vi "Convert Plot Interpolation (PN to List).vi"(8 "Error In":errorcluster, 11 "Plot Interpolation (PN)":u8) -> (0 "Error Out":errorcluster, 3 "Plot Interpolation (List)":T1)   [LabVIEW 2021, in "Graphs.lvlib"]
uses:
  LabVIEW Plot Interpolation.ctl
  Graphs.lvlib
panel:
  # "see the License on the block diagram (Ctrl+E or Window:Show Block Diagram)"
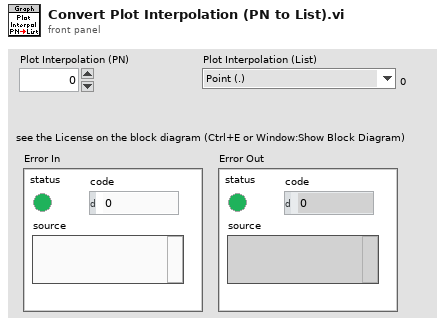
[diagram p1: front panel]
types:
  T1 = typedef "Graphs.lvlib/LabVIEW Plot Interpolation.ctl" = enum16{"Point (.)", "Stepwise Right (--.)", "Line + Point (\\. /)", "Stepwise Left (.--)", "Stepwise Centered (-.-)", "Stepwise Vertical (|.|)", "Line (-)", "Use Previous Plot's Style"}
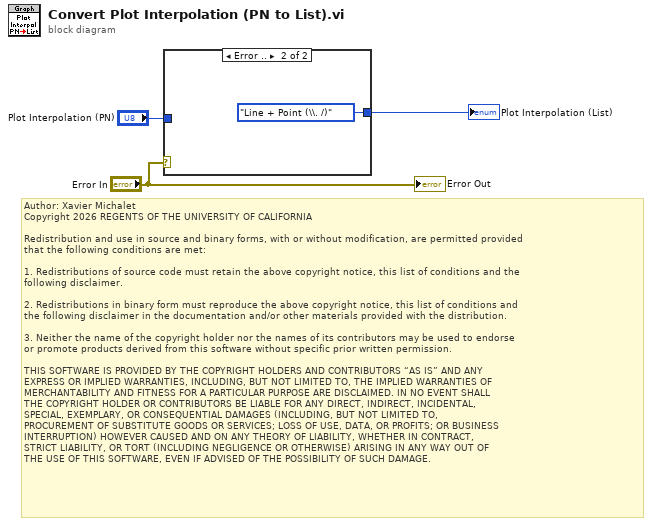
[diagram p0: block diagram]
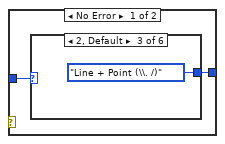
[diagram p2: hidden frame]
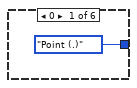
[diagram p3: hidden frame]
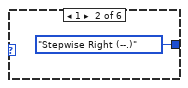
[diagram p4: hidden frame]
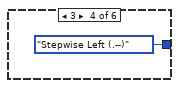
[diagram p5: hidden frame]
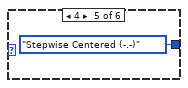
[diagram p6: hidden frame]
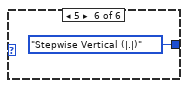
[diagram p7: hidden frame]
diagram:
  # "Author: Xavier Michalet\nCopyright 2026 REGENTS OF THE UNIVERSITY OF CALIFORNIA\n\nRedistribution and use in source and binary forms, with or without modification, are permitted provided\nthat the following conditions are met:\n\n1. Redistributions of source code must retain the above copyright notice, this list of conditions and the\nfollowing disclaimer.\n\n2. Redistributions in binary form must reproduce the above copyright notice, this list of conditions and\nthe following disclaimer in the documentation and/or other materials provided with the distribution.\n\n3. Neither the name of the copyright holder nor the names of its contributors may be used to endorse \nor promote products derived from this software without specific prior written permission.\n\nTHIS SOFTWARE IS PROVIDED BY THE COPYRIGHT HOLDERS AND CONTRIBUTORS “AS IS” AND ANY \nEXPRESS OR IMPLIED WARRANTIES, INCLUDING, BUT NOT LIMITED TO, THE IMPLIED WARRANTIES OF\nMERCHANTABILITY AND FITNESS FOR A PARTICULAR PURPOSE ARE DISCLAIMED. IN NO EVENT SHALL\nTHE COPYRIGHT HOLDER OR CONTRIBUTORS BE LIABLE FOR ANY DIRECT, INDIRECT, INCIDENTAL, \nSPECIAL, EXEMPLARY, OR CONSEQUENTIAL DAMAGES (INCLUDING, BUT NOT LIMITED TO, \nPROCUREMENT OF SUBSTITUTE GOODS OR SERVICES; LOSS OF USE, DATA, OR PROFITS; OR BUSINESS\nINTERRUPTION) HOWEVER CAUSED AND ON ANY THEORY OF LIABILITY, WHETHER IN CONTRACT, \nSTRICT LIABILITY, OR TORT (INCLUDING NEGLIGENCE OR OTHERWISE) ARISING IN ANY WAY OUT OF\nTHE USE OF THIS SOFTWARE, EVEN IF ADVISED OF THE POSSIBILITY OF SUCH DAMAGE."
  n1 = case shown="Error .." "Error In" {
    tunnel: "Plot Interpolation (PN)" -> [w5 _]
    tunnel: [w4 LabVIEW_Plot_Interpolation."Line + Point (\\. /)" ("Plot Interpolation (List)")] -> w1
    frame No Error {
      n2 = case shown="2, Default" w5 {
        tunnel: [LabVIEW_Plot_Interpolation."Point (.)" ("Plot Interpolation (List)") LabVIEW_Plot_Interpolation."Stepwise Right (--.)" ("Plot Interpolation (List)") LabVIEW_Plot_Interpolation."Line + Point (\\. /)" ("Plot Interpolation (List)") LabVIEW_Plot_Interpolation."Stepwise Left (.--)" ("Plot Interpolation (List)") LabVIEW_Plot_Interpolation."Stepwise Centered (-.-)" ("Plot Interpolation (List)") LabVIEW_Plot_Interpolation."Stepwise Vertical (|.|)" ("Plot Interpolation (List)")] -> w4
        frame 0 {
        }
        frame 1 {
        }
        frame 2, Default {
        }
        frame 3 {
        }
        frame 4 {
        }
        frame 5 {
        }
      }
    }
    frame Error {
    }
  }
  "Plot Interpolation (List)" <- w1
  "Error Out" <- "Error In"
